vi "Table_InitFrontPanel.vi"(8 "error in (no error)":errorcluster, 10 "Defer Panel Updates":bool=TRUE, 11 "VI in":refnum<vi>) -> (0 "error out":errorcluster)   [LabVIEW 2012]
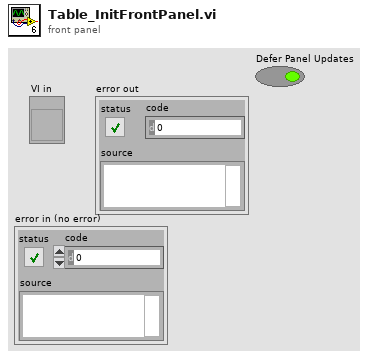
[diagram p1: front panel]
types:
  T1 = enum32{"Invalid", "Standard", "Closed", "Hidden", "Minimized", "Maximized"}
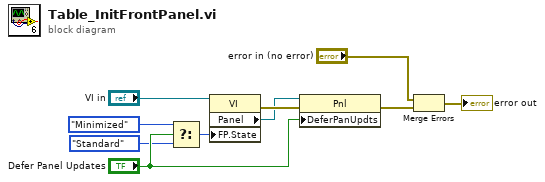
[diagram p0: block diagram]
diagram:
  n1 = Select(t=T1."Minimized" ("Front Panel Window:State"), s="Defer Panel Updates", f=T1."Standard") -> (s? t:f=w4:T1)
  n2 = property class="VI"(reference="VI in", "FP.State"=w4) -> (error out=w9:errorcluster, "Panel"=w8:refnum<vi>)  [unwired: 1 in, 1 out]
  n3 = property class="Pnl"(reference=w8, error in=w9, "DeferPanUpdts"="Defer Panel Updates") -> (error out=w10:errorcluster)  [unwired: 1 out]
  n4 = Merge Errors("error in (no error)", w10) -> (→"error out":errorcluster)
